vi "Coward.vi"(8 "error in (no error)":errorcluster, 10 "Map":i32[](array[numeric]), 11 "Mother In":refnum<class "Formics.lvclass">) -> (0 "error out":errorcluster, 1 "Direction":T1, 2 "Action":T2, 3 "Mother Out":refnum<class "Formics.lvclass">, 4 "Replicated":refnum<class "Square.lvclass">)   [LabVIEW 2015, in "Formics.lvclass"]
uses:
  Formics.lvclass
  Type Defs/Action Enum.ctl
  Type Defs/Direction Enum.ctl
  Square/Square.lvclass
  Formics.lvclass/Formics.ctl
  Attack Options.ctl
  Coward Options.ctl
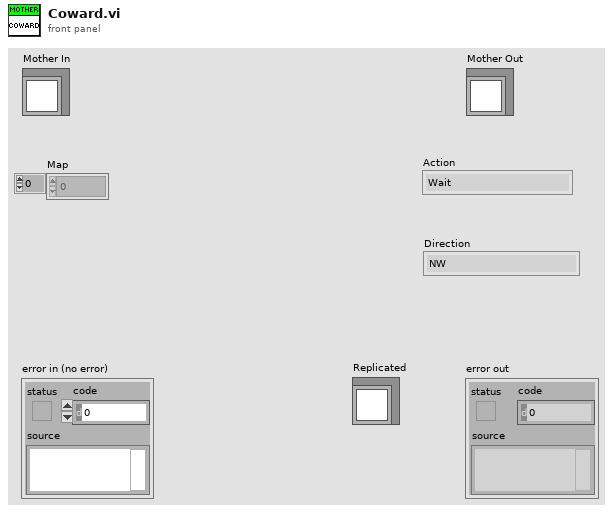
[diagram p1: front panel]
types:
  T1 = typedef "Square.lvclass/Direction Enum.ctl" = enum16{"NW", "N", "NE", "E", "SE", "S", "SW", "W"}
  T2 = typedef "Square.lvclass/Action Enum.ctl" = enum16{"Wait", "Move", "Attack", "Replicate"}
  T3 = typedef "Formics.lvclass/Coward Options.ctl" = enum16{"Default", "Attack behind and continue", "Attack behind and retreat", "Move Back", "Check if still there"}
  T4 = typedef "Formics.lvclass/Attack Options.ctl" = enum16{"Attack", "Run", "Distract"}
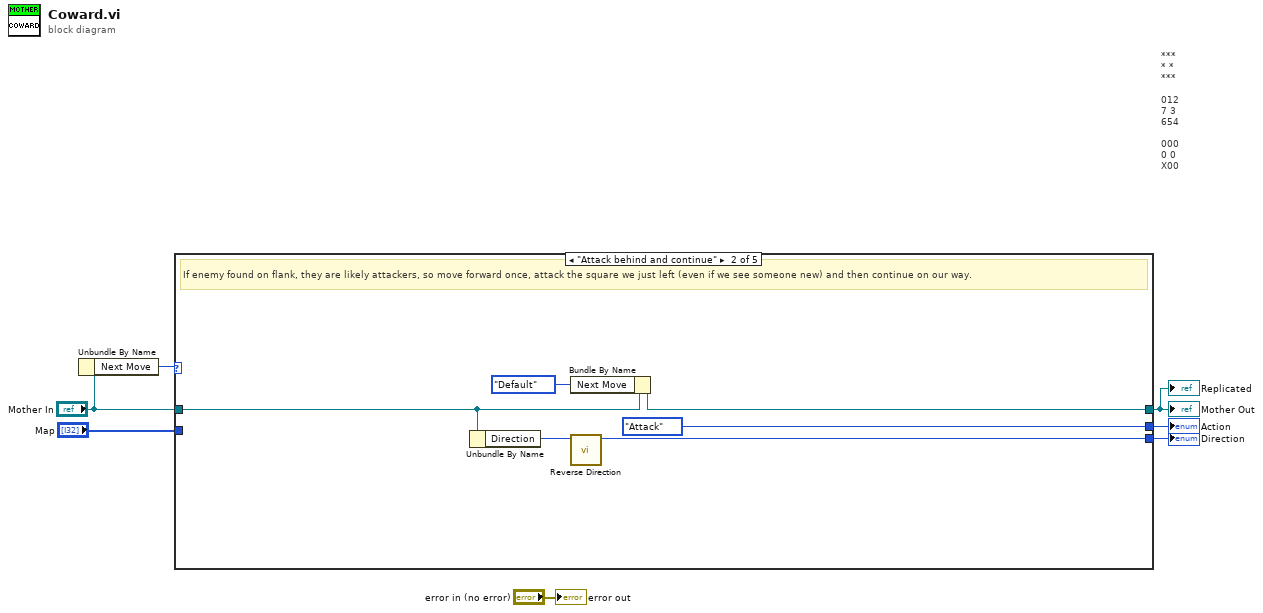
[diagram p0: block diagram]
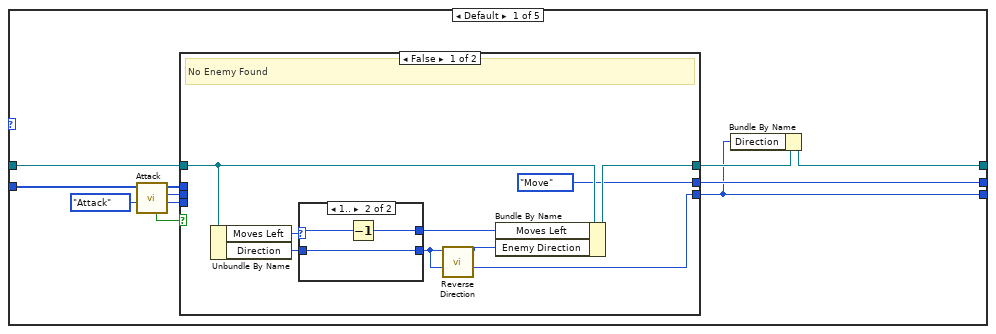
[diagram p2: hidden frame]
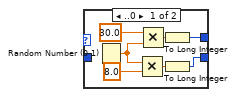
[diagram p3: hidden frame]
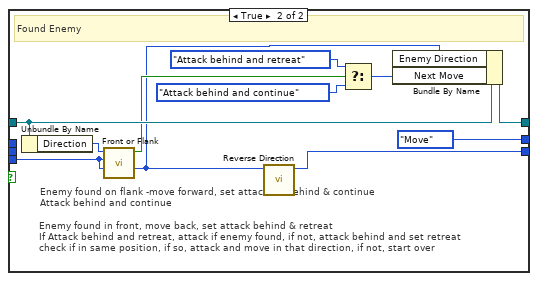
[diagram p4: hidden frame]
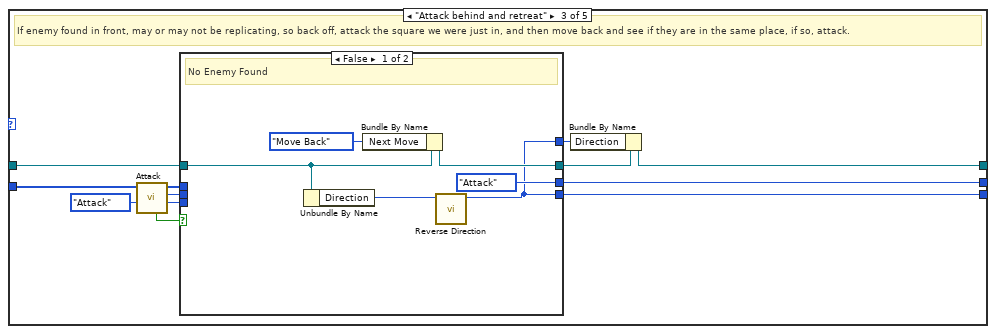
[diagram p5: hidden frame]
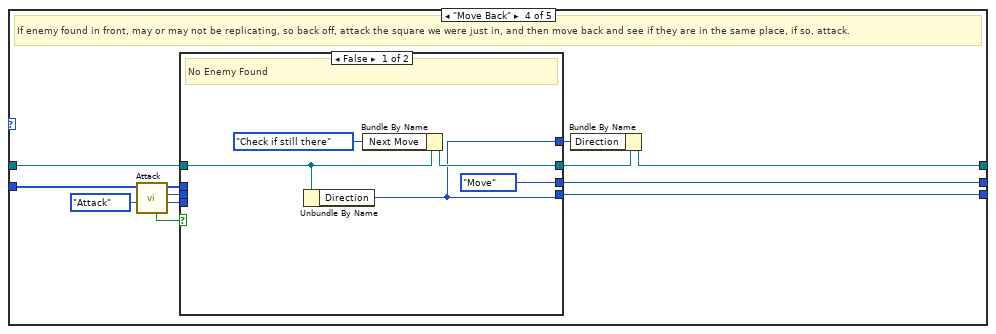
[diagram p7: hidden frame]
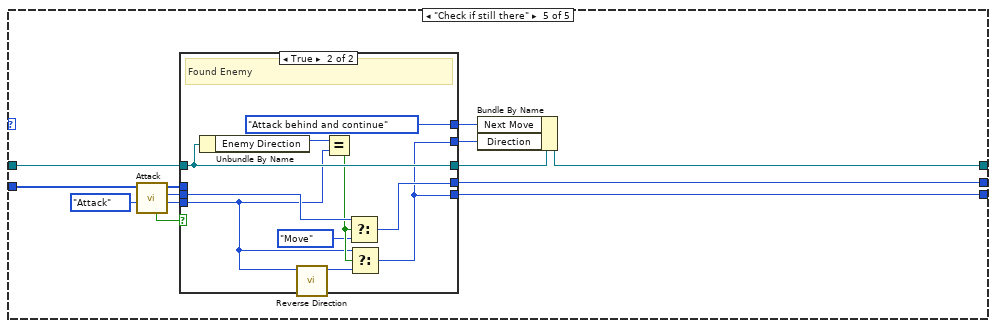
[diagram p9: hidden frame]
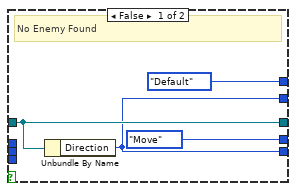
[diagram p10: hidden frame]
diagram:
  # "***\n* *\n***\n\n012\n7 3\n654\n\n000\n0 0\nX00"
  n1 = Unbundle By Name("Mother In") -> ("Next Move"=w1:T3)
  n2 = case shown="\"Attack behind and continue\"" w1 {
    tunnel: [w15 Action_Enum."Attack" ("Action") w61 w82 w103] -> w6
    tunnel: [w8 w51 w59 w80 w101] -> w5
    tunnel: [w9 w50 w54 w75 w96] -> w4
    tunnel: "Map" -> [w11 _ w56 w77 w98]
    tunnel: "Mother In" -> [w10 w47 w55 w76 w97]
    frame Default {
      n3 = call "Attack.vi"("Attack?"=Attack_Options."Attack", "Maze (0: Empty, -1: Enemy. >0: Teammate"=w11) -> ("Direction"=w14:i32, "Action"=w16:T2, "Maze (0: Empty, -1: Enemy. >0: Teammate 2"=w12:i32[], "Enemy Found?"=w17:bool)  [unwired: 4 in, 2 out]
      n4 = case shown="False" w17 {
        tunnel: w16 -> [_ _]
        tunnel: [Action_Enum."Move" ("Action") Action_Enum."Move" ("Action")] -> w15
        tunnel: w14 -> [_ w37]
        tunnel: [w20 w38] -> w8
        tunnel: w12 -> [_ _]
        tunnel: w10 -> [w26 w46]
        tunnel: [w25 w45] -> w13
        frame False {
          # "No Enemy Found"
          n5 = Unbundle By Name(w26) -> ("Moves Left"=w23:i32, "Direction"=w21:i32)
          n6 = case shown="1.." w23 {
            selector: w23 -> [_ w36]
            tunnel: [w28 w35] -> w22
            tunnel: [w27 w34] -> w20
            tunnel: w21 -> [_ w34]
            frame ..0 {
              n7 = Random Number (0-1)() -> (number: 0 to 1=w29:dbl)
              n8 = Multiply(x=w29, y=8.0) -> (x*y=w33:dbl)
              n9 = Multiply(x=30.0 ("t"), y=w29) -> (x*y=w31:dbl)
              n10 = To Long Integer(number=w31) -> (32bit integer=w28:i32)
              n11 = To Long Integer(number=w33) -> (32bit integer=w27:i32)
            }
            frame 1.. {
              n12 = Decrement(x=w36) -> (x-1=w35:i32)
            }
          }
          n13 = call "Reverse Direction.vi"("Direction"=w20) -> ("Numeric"=w19:i32)  [unwired: 10 in]
          n14 = Bundle By Name(cluster=w26, "Moves Left"=w22, "Enemy Direction"=w19) -> (w25:refnum<class "Formics.lvclass">)
        }
        frame True {
          # "Enemy found in front, move back, set attack behind & retreat\nIf Attack behind and retreat, attack if enemy found, if not, attack behind and set retreat\ncheck if in same position, if so, attack and move in that direction, if not, start over"
          # "Enemy found on flank -move forward, set attack for behind & continue\nAttack behind and continue"
          # "Found Enemy"
          n15 = Unbundle By Name(w46) -> ("Direction"=w44:i32)
          n16 = call "Front or Flank.vi"("Enemy Direction"=w37, "Direction"=w44) -> ("Front?"=w43:bool)  [unwired: 9 in]
          n17 = call "Reverse Direction.vi"("Direction"=w37) -> ("Numeric"=w38:i32)  [unwired: 10 in]
          n18 = Select(t=Coward_Options."Attack behind and retreat" ("Next Move"), s=w43, f=Coward_Options."Attack behind and continue" ("Next Move")) -> (s? t:f=w39:T3)
          n19 = Bundle By Name(cluster=w46, "Enemy Direction"=w37, "Next Move"=w39) -> (w45:refnum<class "Formics.lvclass">)
        }
      }
      n20 = Bundle By Name(cluster=w13, "Direction"=w8) -> (w9:refnum<class "Formics.lvclass">)
    }
    frame "Attack behind and continue" {
      # "If enemy found on flank, they are likely attackers, so move forward once, attack the square we just left (even if we see someone new) and then continue on our way."
      n21 = Unbundle By Name(w47) -> ("Direction"=w49:i32)
      n22 = Bundle By Name(cluster=w47, "Next Move"=Coward_Options."Default") -> (w50:refnum<class "Formics.lvclass">)
      n23 = call "Reverse Direction.vi"("Direction"=w49) -> ("Numeric"=w51:i32)  [unwired: 10 in]
    }
    frame "Attack behind and retreat" {
      # "If enemy found in front, may or may not be replicating, so back off, attack the square we were just in, and then move back and see if they are in the same place, if so, attack."
      n24 = call "Attack.vi"("Attack?"=Attack_Options."Attack", "Maze (0: Empty, -1: Enemy. >0: Teammate"=w56) -> ("Direction"=w60:i32, "Action"=w62:T2, "Maze (0: Empty, -1: Enemy. >0: Teammate 2"=w57:i32[], "Enemy Found?"=w63:bool)  [unwired: 4 in, 2 out]
      n25 = case shown="False" w63 {
        tunnel: w62 -> [_ w72]
        tunnel: [Action_Enum."Attack" ("Action") w72] -> w61
        tunnel: w60 -> [_ w71]
        tunnel: [w65 w71] -> w59
        tunnel: w57 -> [_ _]
        tunnel: w55 -> [w69 w73]
        tunnel: [w68 w73] -> w58
        tunnel: [w65 w71] -> w53
        frame False {
          # "No Enemy Found"
          n26 = Unbundle By Name(w69) -> ("Direction"=w66:i32)
          n27 = Bundle By Name(cluster=w69, "Next Move"=Coward_Options."Move Back") -> (w68:refnum<class "Formics.lvclass">)
          n28 = call "Reverse Direction.vi"("Direction"=w66) -> ("Numeric"=w65:i32)  [unwired: 10 in]
        }
        frame True {
          # "If enemy found in front, and then enemy found when moving away, \nattack the second since we are hemmed in and don't \nhave time to attack the square we just left."
          # "Found Enemy"
        }
      }
      n29 = Bundle By Name(cluster=w58, "Direction"=w53) -> (w54:refnum<class "Formics.lvclass">)
    }
    frame "Move Back" {
      # "If enemy found in front, may or may not be replicating, so back off, attack the square we were just in, and then move back and see if they are in the same place, if so, attack."
      n30 = call "Attack.vi"("Attack?"=Attack_Options."Attack", "Maze (0: Empty, -1: Enemy. >0: Teammate"=w77) -> ("Direction"=w81:i32, "Action"=w83:T2, "Maze (0: Empty, -1: Enemy. >0: Teammate 2"=w78:i32[], "Enemy Found?"=w84:bool)  [unwired: 4 in, 2 out]
      n31 = case shown="False" w84 {
        tunnel: w83 -> [_ w92]
        tunnel: [Action_Enum."Move" ("Action") w92] -> w82
        tunnel: w81 -> [_ w91]
        tunnel: [w86 w91] -> w80
        tunnel: w78 -> [_ _]
        tunnel: w76 -> [w89 w93]
        tunnel: [w88 w93] -> w79
        tunnel: [w86 w91] -> w74
        frame False {
          # "No Enemy Found"
          n32 = Unbundle By Name(w89) -> ("Direction"=w86:i32)
          n33 = Bundle By Name(cluster=w89, "Next Move"=Coward_Options."Check if still there") -> (w88:refnum<class "Formics.lvclass">)
        }
        frame True {
          # "If enemy appears, attack it."
          # "Found Enemy"
        }
      }
      n34 = Bundle By Name(cluster=w79, "Direction"=w74) -> (w75:refnum<class "Formics.lvclass">)
    }
    frame "Check if still there" {
      n35 = call "Attack.vi"("Attack?"=Attack_Options."Attack", "Maze (0: Empty, -1: Enemy. >0: Teammate"=w98) -> ("Direction"=w102:i32, "Action"=w104:T2, "Maze (0: Empty, -1: Enemy. >0: Teammate 2"=w99:i32[], "Enemy Found?"=w105:bool)  [unwired: 4 in, 2 out]
      n36 = case shown="True" w105 {
        tunnel: w104 -> [_ w117]
        tunnel: [Action_Enum."Move" ("Action") w114] -> w103
        tunnel: w102 -> [_ w112]
        tunnel: [w108 w111] -> w101
        tunnel: w99 -> [_ _]
        tunnel: w97 -> [w109 w120]
        tunnel: [w109 w120] -> w100
        tunnel: [w108 w111] -> w95
        tunnel: [Coward_Options."Default" ("Next Move") Coward_Options."Attack behind and continue" ("Next Move")] -> w94
        frame False {
          # "No Enemy Found"
          n37 = Unbundle By Name(w109) -> ("Direction"=w108:i32)
        }
        frame True {
          # "Found Enemy"
          n38 = Unbundle By Name(w120) -> ("Enemy Direction"=w119:i32)
          n39 = call "Reverse Direction.vi"("Direction"=w112) -> ("Numeric"=w115:i32)  [unwired: 10 in]
          n40 = Equal?(x=w119, y=w112) -> (x = y?=w116:bool)
          n41 = Select(t=w117, s=w116, f=Action_Enum."Move") -> (s? t:f=w114:T2)
          n42 = Select(t=w112, s=w116, f=w115) -> (s? t:f=w111:i32)
        }
      }
      n43 = Bundle By Name(cluster=w100, "Next Move"=w94, "Direction"=w95) -> (w96:refnum<class "Formics.lvclass">)
    }
  }
  "Mother Out" <- w4
  "Action" <- w6
  "Direction" <- w5
  "Replicated" <- w4
  "error out" <- "error in (no error)"
